vi "Microscopy.acqEngineEncodeEdge.vi"(9 "Early RefTrig?":bool, 10 "Later RefTrig?":bool) -> (1 "Trig Offset":u8, 2 "Send RefTrig":bool)   [LabVIEW 2011]
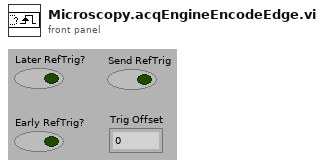
[diagram p1: front panel]
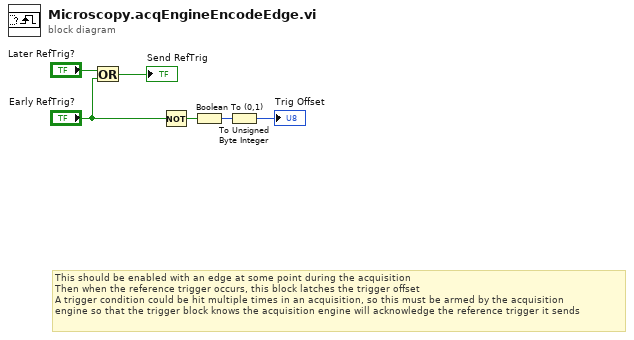
[diagram p0: block diagram]
diagram:
  # "This should be enabled with an edge at some point during the acquisition\nThen when the reference trigger occurs, this block latches the trigger offset\nA trigger condition could be hit multiple times in an acquisition, so this must be armed by the acquisition\nengine so that the trigger block knows the acquisition engine will acknowledge the reference trigger it sends"
  n1 = Or(x="Later RefTrig?", y="Early RefTrig?") -> (x .or. y?=→"Send RefTrig":bool)
  n2 = Not(x="Early RefTrig?") -> (.not. x?=w6:bool)
  n3 = Boolean To (0,1)(Boolean=w6) -> (0, 1=w5:i16)
  n4 = To Unsigned Byte Integer(number=w5) -> (unsigned 8bit integer=→"Trig Offset":u8)
